vi "GBL System.vi"() -> ()   [LabVIEW 2017]
doc: "Developed by Kevin Thompson\nkevin@thompsonengineering.net\n\nCopyright 2018-2020\nThompson Engineering, LLC"
panel:
  in  "AppVersion":string
  out "RunTimeSys?":bool
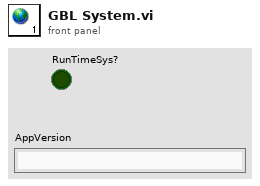
[diagram p1: front panel]
diagram:
